vi "Swerve Auton.vi"(8 "Heading":dbl=270.0, 9 "y Distance":dbl=50.0, 10 "x Distance":dbl=-40.0, 11 "Power":dbl=0.5) -> ()   [LabVIEW 2019]
uses:
  Robot Global Data.vi
  <vilib>/addons/control/pid/pid.llb/PID (DBL).vi
  <vilib>/addons/control/pid/NI_PID_pid.lvlib
panel:
  in  "PID gains X":T1={"proportional gain (Kc)"=0.04, "integral time (Ti, min)"=0.0, "derivative time (Td, min)"=0.0} {"derivative time (Td, min)" format="%.3f"; "integral time (Ti, min)" format="%.3f"; "proportional gain (Kc)" format="%.3f"}
  in  "PID gains Y":T1={"proportional gain (Kc)"=0.04, "integral time (Ti, min)"=0.0, "derivative time (Td, min)"=0.0} {"derivative time (Td, min)" format="%.3f"; "integral time (Ti, min)" format="%.3f"; "proportional gain (Kc)" format="%.3f"}
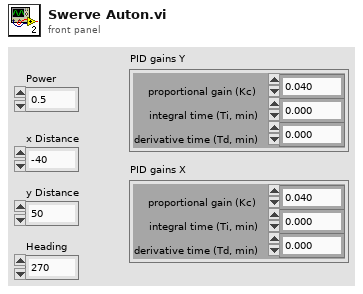
[diagram p1: front panel]
types:
  T1 = cluster{"proportional gain (Kc)":dbl, "integral time (Ti, min)":dbl, "derivative time (Td, min)":dbl}
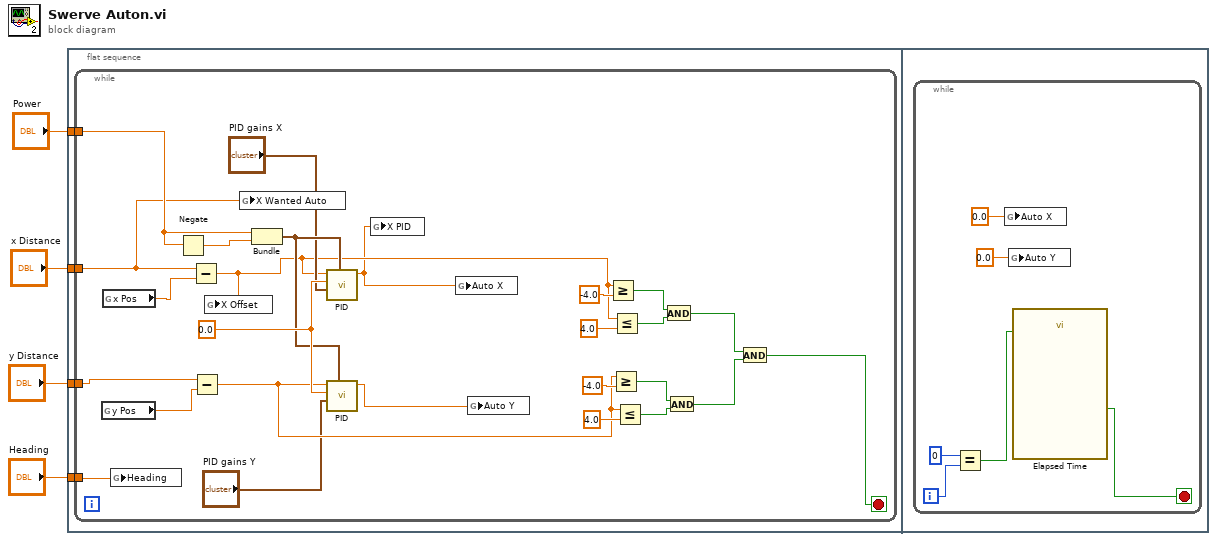
[diagram p0: block diagram]
diagram:
  n1 = flat-sequence {
    tunnel: "Power" -> [w5]
    tunnel: "x Distance" -> [w6]
    tunnel: "y Distance" -> [w7]
    tunnel: "Heading" -> [w8]
    frame #0 {
      n2 = while {
        tunnel: w8 -> [w34]
        tunnel: w7 -> [w33]
        tunnel: w6 -> [w11]
        tunnel: w5 -> [w29]
        stop <- w16 stop-if-true
        w31 = 0.0 ("process variable")
        n3 = global read "Robot Global Data.vi" "y Pos"() -> (w32:dbl)
        n4 = global read "Robot Global Data.vi" "x Pos"() -> (w13:dbl)
        n5 = global write "Robot Global Data.vi" "Heading"(w34) -> ()
        n6 = Negate(x=w29) -> (-x=w30:dbl)
        n7 = Subtract(x=w11, y=w13) -> (x-y=w10:dbl)
        n8 = Subtract(x=w33, y=w32) -> (x-y=w17:dbl)
        n9 = global write "Robot Global Data.vi" "X Offset"(w10) -> ()
        n10 = global write "Robot Global Data.vi" "X Wanted Auto"(w11) -> ()
        n11 = Bundle("Power"=w29, w30) -> (w28:cluster{"Power":dbl, dbl})  [unwired: 1 in]
        n12 = call-poly <vilib>:"PID.vi"("output range"=w28, "PID gains"="PID gains X", "process variable"=w31, "setpoint"=w10) -> ("output"=w9:dbl)  [unwired: 6 in, 1 out]
        n13 = call-poly <vilib>:"PID.vi"("output range"=w28, "PID gains"="PID gains Y", "process variable"=w31, "setpoint"=w17) -> ("output"=w12:dbl)  [unwired: 6 in, 1 out]
        n14 = global write "Robot Global Data.vi" "X PID"(w9) -> ()
        n15 = global write "Robot Global Data.vi" "Auto X"(w9) -> ()
        n16 = global write "Robot Global Data.vi" "Auto Y"(w12) -> ()
        n17 = Greater Or Equal?(x=w10, y=-4.0) -> (x >= y?=w24:bool)
        n18 = Greater Or Equal?(x=w17, y=-4.0) -> (x >= y?=w19:bool)
        n19 = Less Or Equal?(x=w10, y=4.0) -> (x <= y?=w27:bool)
        n20 = Less Or Equal?(x=w17, y=4.0) -> (x <= y?=w22:bool)
        n21 = And(x=w24, y=w27) -> (x .and. y?=w23:bool)
        n22 = And(x=w19, y=w22) -> (x .and. y?=w18:bool)
        n23 = And(x=w23, y=w18) -> (x .and. y?=w16:bool)
      }
    }
    frame #1 {
      n24 = while {
        i -> [w38]
        stop <- w36 stop-if-true
        n25 = Equal?(x=0, y=w38) -> (x = y?=w35:bool)
        n26 = global write "Robot Global Data.vi" "Auto X"(0.0 ("Auto X")) -> ()
        n27 = global write "Robot Global Data.vi" "Auto Y"(0.0 ("Auto Y")) -> ()
        n28 = call "Elapsed Time"("Reset"=w35) -> ("Time has Elapsed"=w36:bool)  [unwired: 11 in, 7 out]
      }
    }
  }
